vi "Case structures.vi"() -> ()   [LabVIEW 2021]
panel:
  in  "Enum":enum16{"Plus\n", "Minus\n", "Multiply"}(ring)
  out "Numeric 3":dbl
  in  "Numeric 2":dbl
  in  "Numeric":dbl
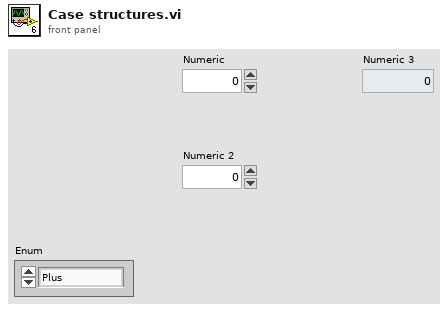
[diagram p1: front panel]
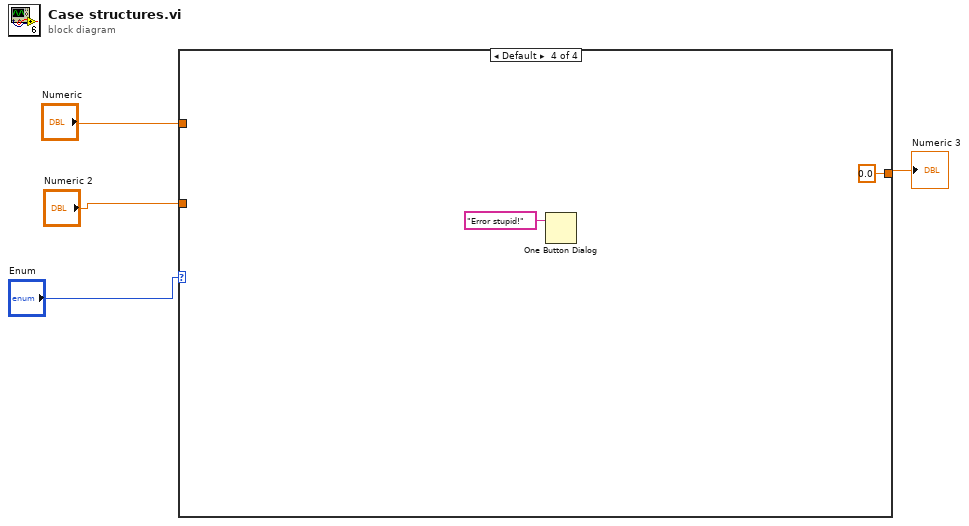
[diagram p0: block diagram]
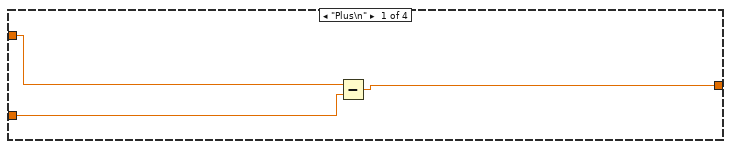
[diagram p2: hidden frame]
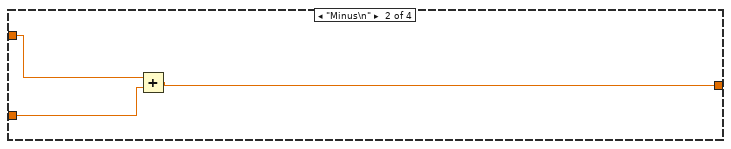
[diagram p3: hidden frame]
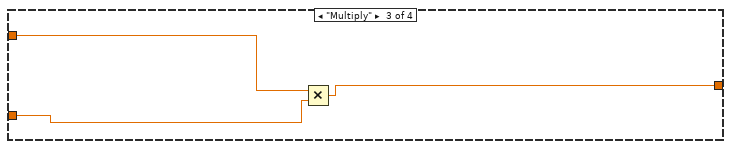
[diagram p4: hidden frame]
diagram:
  n1 = case shown="Default" "Enum" {
    tunnel: "Numeric" -> [w7 w10 w13 _]
    tunnel: "Numeric 2" -> [w6 w9 w12 _]
    tunnel: [w5 w8 w11 0.0] -> w2
    frame "Plus\n" {
      n2 = Subtract(x=w7, y=w6) -> (x-y=w5:dbl)
    }
    frame "Minus\n" {
      n3 = Add(x=w10, y=w9) -> (x+y=w8:dbl)
    }
    frame "Multiply" {
      n4 = Multiply(x=w13, y=w12) -> (x*y=w11:dbl)
    }
    frame Default {
      n5 = One Button Dialog(message="Error stupid!") -> ()  [unwired: 1 in, 1 out]
    }
  }
  "Numeric 3" <- w2
